vi "Write TSP Link Synchronization Line Data.vi"(5 "Mask (0)":i32, 6 "Port (0)":i32, 7 "Bit (0: Low)":i32(ring) items=["Low", "High"], 8 "error in (no error)":errorcluster, 9 "TSP Link Line (1)":i32=1, 10 "Data Type (0: Bit)":i32(ring) items=["Bit", "Port", "Mask"], 11 "VISA resource name":refnum<visa-resource-name>) -> (0 "error out":errorcluster, 3 "VISA resource name out":refnum<visa-resource-name>)   [LabVIEW 2017, in "Keithley 2600 Series.lvlib"]
doc: "Write data to TSP-Link synchronization line.\n\n<b>Note:</b>\nThis VI is not available on models 2604B, 2614B, 2634B."
uses:
  <instrlib>/Keithley 2600 Series/Keithley 2600 Series.lvlib
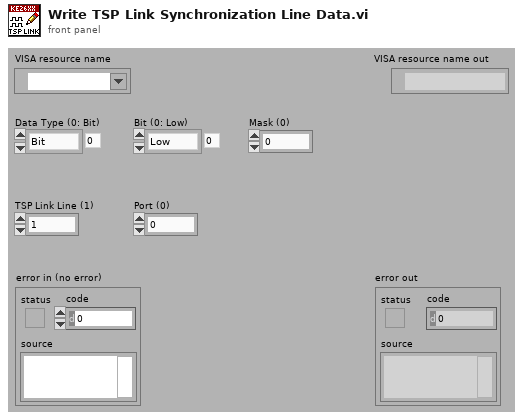
[diagram p1: front panel]
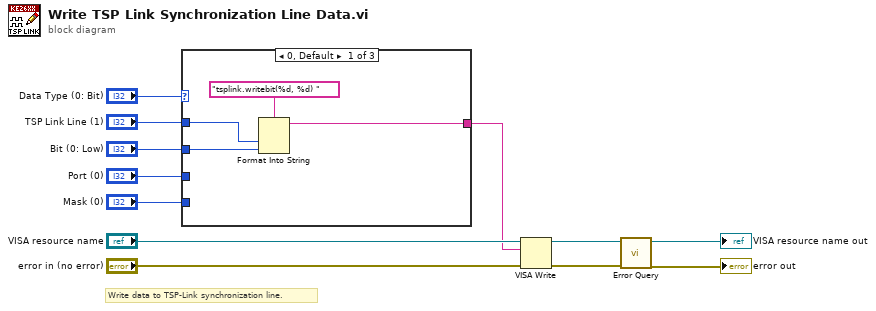
[diagram p0: block diagram]
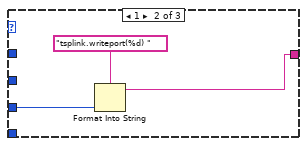
[diagram p2: hidden frame]
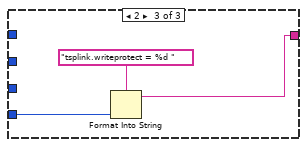
[diagram p3: hidden frame]
diagram:
  # "Write data to TSP-Link synchronization line."
  n1 = case shown="0, Default" "Data Type (0: Bit)" {
    tunnel: "TSP Link Line (1)" -> [w15 _ _]
    tunnel: "Bit (0: Low)" -> [w14 _ _]
    tunnel: [w13 w17 w20] -> w3
    tunnel: "Port (0)" -> [_ w18 _]
    tunnel: "Mask (0)" -> [_ _ w21]
    frame 0, Default {
      n2 = Format Into String(format string="tsplink.writebit(%d, %d) ", w15, w14) -> (resulting string=w13:string)  [unwired: 2 in, 1 out]
    }
    frame 1 {
      n3 = Format Into String(format string="tsplink.writeport(%d) ", w18) -> (resulting string=w17:string)  [unwired: 2 in, 1 out]
    }
    frame 2 {
      n4 = Format Into String(format string="tsplink.writeprotect = %d ", w21) -> (resulting string=w20:string)  [unwired: 2 in, 1 out]
    }
  }
  n5 = VISA Write(VISA resource name="VISA resource name", write buffer=w3, error in (no error)="error in (no error)") -> (VISA resource name out=w10:refnum<visa-resource-name>, error out=w9:errorcluster)  [unwired: 1 out]
  n6 = call <instrlib>:"Error Query.vi"("error in (no error)"=w9, "VISA resource name"=w10) -> ("error out"=→"error out":errorcluster, "VISA resource name out"=→"VISA resource name out":refnum<visa-resource-name>)  [unwired: 6 in, 2 out]
